vi "Logging_Singleton_Example.vi"() -> ()   [LabVIEW 2024]
uses:
  Stream/Writer/DETT/DETTWriter.lvclass
  C:/Git/JA/JQMH/RQMHCore/Stream/INetworkWriter/INetworkWriter.lvclass
  LogFormatter/Default/DefaultLogFormat.lvclass
  C:/Git/JA/JQMH/RQMHCore/ErrorReporting/LogFormatter/Interface/ILogFormatter.lvclass
  LogHandle/Event/EventLogHandle.lvclass/EventLogHandle.ctl
  Record/LogRecord.lvclass/LogRecord.ctl
  LogHandle/Stream/StreamLogHandle.lvclass
  C:/Git/JA/JQMH/RQMHCore/ErrorReporting/LogHandle/Interface/LoggingHandle.lvclass
  Stream/ConsoleWriter/ConsoleWriter.lvclass
  LogHandle/Event/EventLogHandle.lvclass
  Record/LogRecord.lvclass
  RQMHLogger/Logger.lvclass
  HandleHolder/HandleHolder.lvclass
  Singleton/LogSingleton.lvlib
  Shared/Level.ctl
  Shared/LoggerShared.lvlib
panel:
  in  "stop":bool
  out "error out":errorcluster
  out "Level":T1
  out "Source":string
  out "Message":string
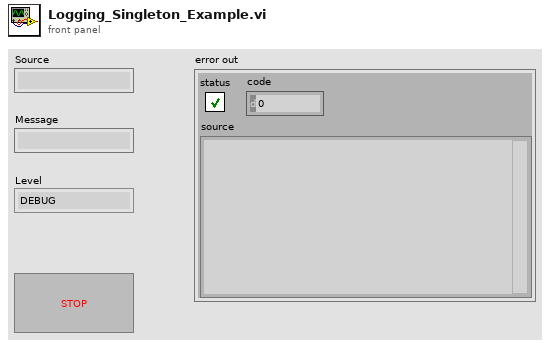
[diagram p1: front panel]
types:
  T1 = typedef "LoggerShared.lvlib/Level.ctl" = enum16{"DEBUG", "INFO", "WARNING", "ERROR", "CRITICAL"}
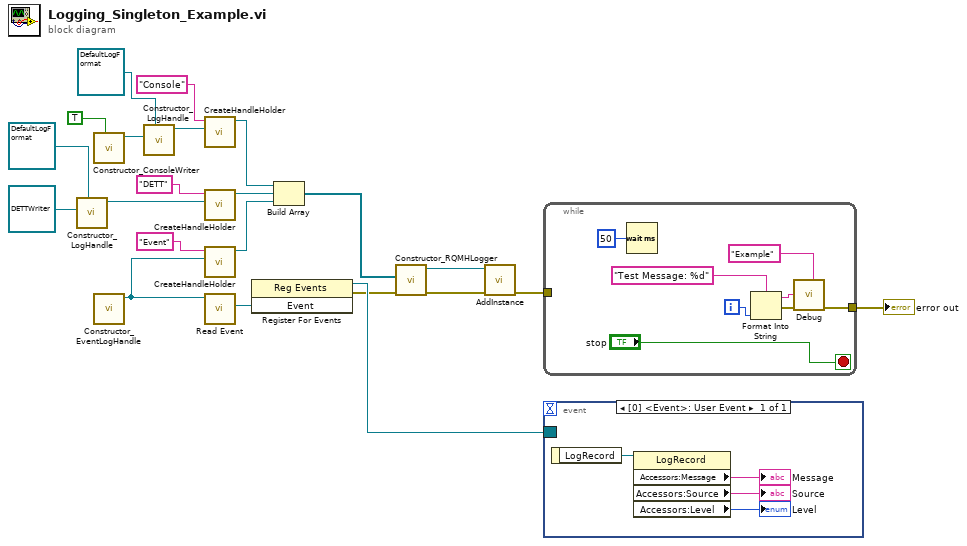
[diagram p0: block diagram]
diagram:
  n1 = call "Constructor_LogHandle.vi"("Formatter"=refnum<class "DefaultLogFormat.lvclass"> refnum ("DefaultLogFormat.lvclass"), "INetworkWriter"=refnum<class "DETTWriter.lvclass"> refnum ("DETTWriter.lvclass")) -> ("FileHandler out"=w12:refnum<class "StreamLogHandle.lvclass">)  [unwired: 8 in, 1 out]
  n2 = call "Constructor_ConsoleWriter.vi"("Autoshow? (f)"=TRUE) -> ("ConsoleWriter out"=w6:refnum<class "ConsoleWriter.lvclass">)  [unwired: 9 in, 1 out]
  n3 = call "Constructor_EventLogHandle.vi"() -> ("EventHandle"=w19:refnum<class "EventLogHandle.lvclass">)  [unwired: 10 in, 1 out]
  n4 = call "Constructor_LogHandle.vi"("Formatter"=refnum<class "DefaultLogFormat.lvclass"> refnum ("DefaultLogFormat.lvclass"), "INetworkWriter"=w6) -> ("FileHandler out"=w10:refnum<class "StreamLogHandle.lvclass">)  [unwired: 8 in, 1 out]
  n5 = call "CreateHandleHolder.vi"("Handle"=w10, "Name"="Console") -> ("HandleHolder out"=w7:refnum<class "HandleHolder.lvclass">)  [unwired: 9 in]
  n6 = call "CreateHandleHolder.vi"("Handle"=w12, "Name"="DETT") -> ("HandleHolder out"=w14:refnum<class "HandleHolder.lvclass">)  [unwired: 9 in]
  n7 = call "CreateHandleHolder.vi"("Handle"=w19, "Name"="Event") -> ("HandleHolder out"=w21:refnum<class "HandleHolder.lvclass">)  [unwired: 9 in]
  n8 = call "Read Event.vi"("EventLogHandle in"=w19) -> ("Event"=w18:refnum<user-event>)  [unwired: 8 in, 2 out]
  n9 = register-events(w18) -> (reference out=w17:refnum<event-registration>, error out=w16:errorcluster)  [unwired: 2 in]
  n10 = Build Array(w7, w14, w21) -> (w20:refnum<class "HandleHolder.lvclass">[])
  n11 = call "Constructor_RQMHLogger.vi"("error in (no error)"=w16, "Handles"=w20) -> ("error out"=w2:errorcluster, "RQMHLogger out"=w3:refnum<class "Logger.lvclass">)  [unwired: 8 in]
  n12 = call "AddInstance.vi"("error in (no error)"=w2, "RQMHLogger in"=w3) -> ("error out"=w1:errorcluster)  [unwired: 9 in]
  n13 = while {
    tunnel: [w23] -> w4
    tunnel: w1 -> [_]
    i -> [w29]
    stop <- "stop" stop-if-true
    n14 = Wait (ms)(milliseconds to wait=u32 50) -> ()  [unwired: 1 out]
    n15 = Format Into String(format string="Test Message: %d" ("Message"), w29) -> (resulting string=w24:string, error out=w27:errorcluster)  [unwired: 2 in]
    n16 = call "Debug.vi"("Source"="Example", "Message"=w24, "error in (no error)"=w27) -> ("error out"=w23:errorcluster)  [unwired: 8 in]
  }
  "error out" <- w4
  n17 = event shown="[0] <Event>: User Event" {
    selector: w17 -> [_]
    dyn-events: _ -> [_]
    timeout: _ -> [_]
    event User Event {
      n18 = event-data() -> ("LogRecord"=w34:refnum<class "LogRecord.lvclass">)  [unwired: 1 in]
      n19 = property class="LogRecord"(reference=w34) -> ("Accessors:Message"=→"Message":string, "Accessors:Source"=→"Source":string, "Accessors:Level"=→"Level":T1)  [unwired: 1 in, 2 out]
    }
  }
